vi "Format As String.vi"(11 "UUID.lvclass":refnum<class "UUID.lvclass">) -> (2 "String":string)   [LabVIEW 2015, in "UUID.lvclass"]
uses:
  UUID.lvclass
  UUID.lvclass/UUID.ctl
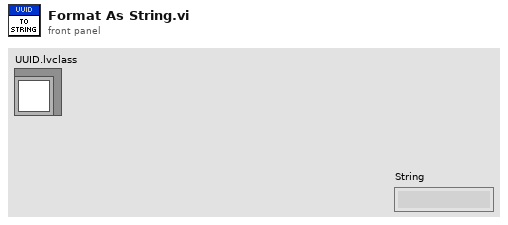
[diagram p1: front panel]
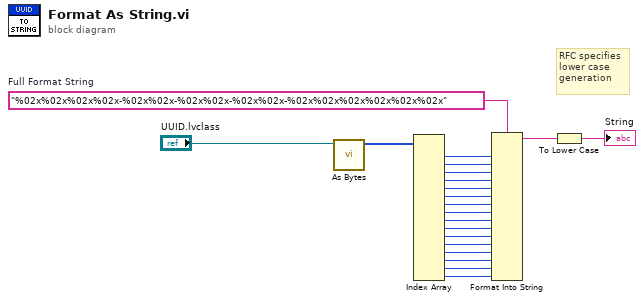
[diagram p0: block diagram]
diagram:
  w19 = "%02x%02x%02x%02x-%02x%02x-%02x%02x-%02x%02x-%02x%02x%02x%02x%02x%02x"  # Full Format String
  # "RFC specifies\nlower case \ngeneration"
  n1 = call "As Bytes.vi"("UUID in"="UUID.lvclass") -> ("Bytes"=w20:u8[])  [unwired: 10 in]
  n2 = Index Array(array=w20) -> (element #1=w18:u8, element #2=w17:u8, element #3=w16:u8, element #4=w15:u8, element #5=w14:u8, element #6=w13:u8, element #7=w12:u8, element #8=w11:u8, element #9=w10:u8, element #10=w9:u8, element #11=w8:u8, element #12=w7:u8, element #13=w6:u8, element #14=w5:u8, element #15=w4:u8, element #16=w3:u8)  [unwired: 16 in]
  n3 = Format Into String(format string=w19, w18, w17, w16, w15, w14, w13, w12, w11, w10, w9, w8, w7, w6, w5, w4, w3) -> (resulting string=w2:string)  [unwired: 2 in, 1 out]
  n4 = To Lower Case(string=w2) -> (all lower case string=→"String":string)
